vi "外观 1.vi"(0 "Data In":T5={"启动"=FALSE, "控制命令"=enum."加标回收（启动采配水）", "测量参数"={"氨氮"=TRUE, "总磷"=TRUE, "总氮"=TRUE, "CODMn"=TRUE, "CODCr"=FALSE}} caption="数据输入", 2 "Display State In":T2={"仪器状态"=FALSE, "仪器时间"=timestamp(0 s since 1904-01-01), "测量参数"={"氨氮"=TRUE, "总磷"=TRUE, "总氮"=TRUE, "CODMn"=TRUE, "CODCr"=FALSE}, "调用模块名称"="", "测试状态"={"启动时间"=timestamp(0 s since 1904-01-01), "结束时间"=timestamp(0 s since 1904-01-01), "启动次数"=0.0}} caption="显示状态输入", 3 "Container State":T4 caption="容器状态") -> (6 "Data Out":T5={"启动"=FALSE, "控制命令"=enum."加标回收（启动采配水）", "测量参数"={"氨氮"=TRUE, "总磷"=TRUE, "总氮"=TRUE, "CODMn"=TRUE, "CODCr"=FALSE}} caption="数据输出", 7 "Display State Out":T2={"仪器状态"=FALSE, "仪器时间"=timestamp(0 s since 1904-01-01), "测量参数"={"氨氮"=TRUE, "总磷"=TRUE, "总氮"=TRUE, "CODMn"=TRUE, "CODCr"=FALSE}, "调用模块名称"="", "测试状态"={"启动时间"=timestamp(0 s since 1904-01-01), "结束时间"=timestamp(0 s since 1904-01-01), "启动次数"=0.0}} caption="显示状态输出", 8 "Action":T1 caption="动作")   [LabVIEW 2016, in "ZK定时设置.xctl"]
uses:
  <vilib>/_xctls/Container State.ctl
  <vilib>/_xctls/Action.ctl
  <vilib>/_xctls/XControlSupport.lvlib
panel:
  in  "周期设置":bool
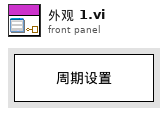
[diagram p1: front panel]
types:
  T1 = typedef "XControlSupport.lvlib/Action.ctl" = cluster{"Data Changed?":bool, "State Changed?":bool, "Action Name":string}
  T2 = typedef "ZK定时设置.xctl/状态 1.ctl" = cluster{"仪器状态":bool, "仪器时间":timestamp, "测量参数":T3, "调用模块名称":string, "测试状态":cluster{"启动时间":timestamp, "结束时间":timestamp, "启动次数":dbl}}
  T3 = typedef "ZK定时设置.xctl/测量参数.ctl" = cluster{"氨氮":bool, "总磷":bool, "总氮":bool, "CODMn":bool, "CODCr":bool}
  T4 = typedef "XControlSupport.lvlib/Container State.ctl" = cluster{"Indicator?":bool, "Run Mode?":bool, " Refnum":refnum<vi>}
  T5 = typedef "ZK定时设置.xctl/数据 1.ctl" = cluster{"启动":bool, "控制命令":T6, "测量参数":T3}
  T6 = typedef "ZK定时设置.xctl/国标控制命令.ctl" = enum16{"加标回收（启动采配水）", "加标回收（不启动采配水）", "水样测试（启动采配水）", "水样测试（不启动采配水）", "平行样测试（启动采配水）", "平行样测试（不启动采配水）", "集成干预测试"}
  T7 = cluster{"启动时间":timestamp, "结束时间":timestamp, "启动次数":dbl}
  T8 = typedef "ZK定时设置.xctl/周期模式设置.ctl" = enum16{"不启用", "定点模式", "间隔模式"}
  T9 = typedef "ZK定时设置.xctl/定点周期设置.ctl" = cluster{"启动命令":T10, "启动命令 2":T10, "启动命令 3":T10, "启动命令 4":T10, "启动命令 5":T10, "启动命令 6":T10, "启动命令 7":T10, "启动命令 8":T10, "启动命令 9":T10, "启动命令 10":T10, "启动命令 11":T10, "启动命令 12":T10, "启动命令 13":T10, "启动命令 14":T10, "启动命令 15":T10, "启动命令 16":T10, "启动命令 17":T10, "启动命令 18":T10, "启动命令 19":T10, "启动命令 20":T10, "启动命令 21":T10, "启动命令 22":T10, "启动命令 23":T10, "启动命令 24":T10}
  T10 = typedef "ZK定时设置.xctl/启动命令选择.ctl" = enum16{"", "加标回收（启动采配水）", "加标回收（不启动采配水）", "水样测试（启动采配水）", "水样测试（不启动采配水）", "平行样测试（启动采配水）", "平行样测试（不启动采配水）", "集成干预测试"}
  T11 = typedef "ZK定时设置.xctl/间隔启动设置.ctl" = cluster{"启动命令":T10, "启动间隔":dbl, "启动次数":i32}
  T12 = cluster{"周期模式":T8, "测量参数":T3, "定点周期":T9, "间隔设置":cluster{"启动命令":T10, "启动间隔":dbl, "启动次数":i32}}
  T13 = cluster{"周期模式":T8, "测量参数":T3, "定点周期":T9, "间隔启动":T11}
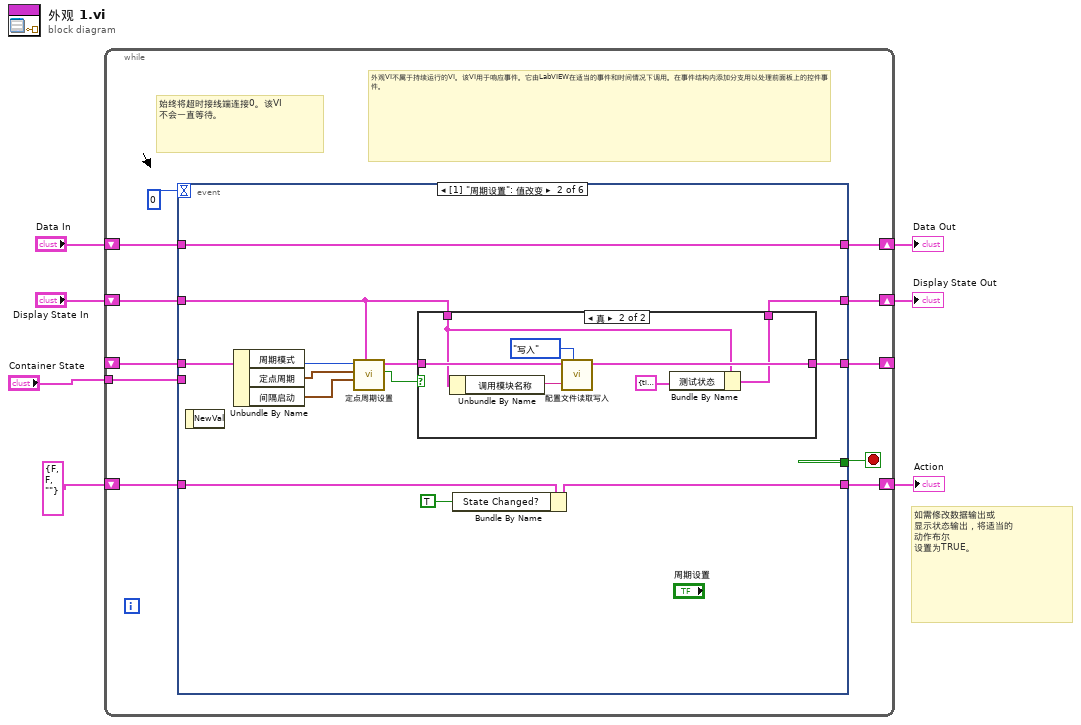
[diagram p0: block diagram]
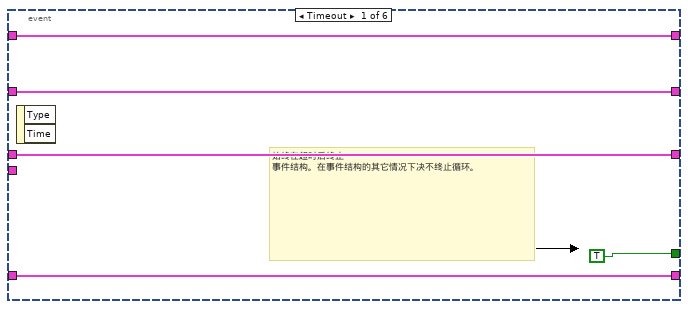
[diagram p2: hidden frame]
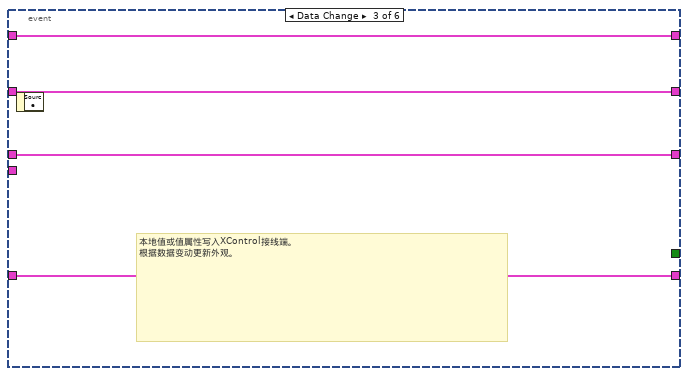
[diagram p4: hidden frame]
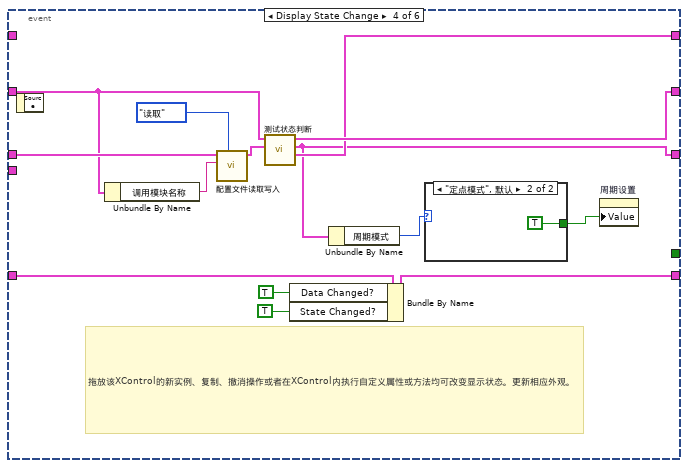
[diagram p5: hidden frame]
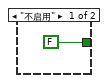
[diagram p6: hidden frame]
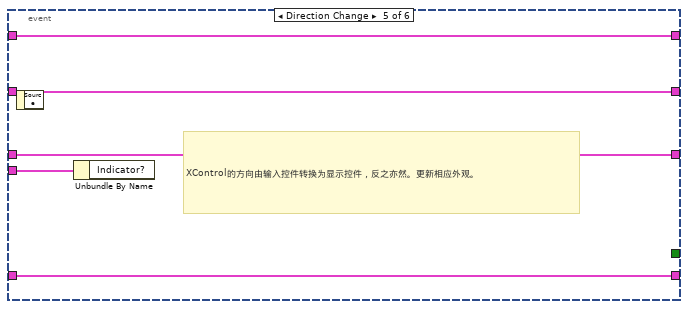
[diagram p7: hidden frame]
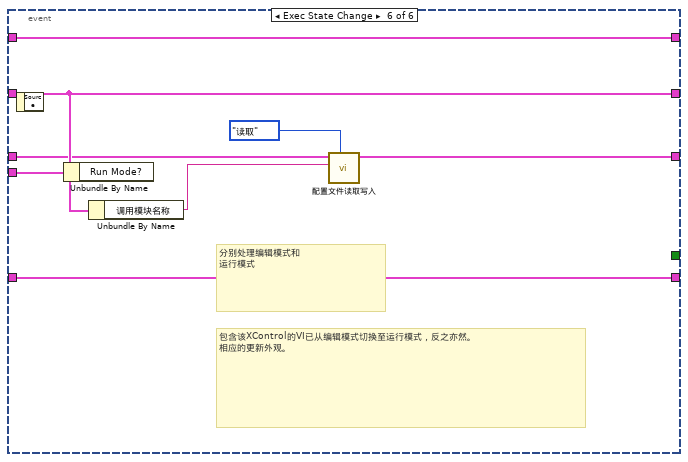
[diagram p8: hidden frame]
diagram:
  # "如需修改数据输出或\n显示状态输出，将适当的\n动作布尔\n设置为TRUE。"
  n1 = while {
    shift-right: [w17] -> w4
    shift-left: "Display State In" -> [w18]
    tunnel: "Container State" -> [w14]
    shift-right: [w12] -> w7
    shift-left: "Data In" -> [w13]
    shift-right: [w10] -> w2
    shift-left: T1 {"Data Changed?"=FALSE, "State Changed?"=FALSE, "Action Name"=""} ("Action") -> [w11]
    shift-right: [w9] -> _
    shift-left: _ -> [w8]
    stop <- w16 stop-if-true
    # "外观VI不属于持续运行的VI。该VI用于响应事件。它由LabVIEW在适当的事件和时间情况下调用。在事件结构内添加分支用以处理前面板上的控件事件。"
    # "始终将超时接线端连接0。该VI\n不会一直等待。"
    n2 = event shown="[1] \"周期设置\": 值改变" {
      selector: _ -> [_ _ _ _ _ _]
      dyn-events: _ -> [_ _ _ _ _ _]
      timeout: 0 -> [_ _ _ _ _ _]
      tunnel: w18 -> [w21 w27 w48 w57 w69 w75]
      tunnel: [w21 w26 w48 w56 w69 w75] -> w17
      tunnel: [TRUE _ _ _ _ _] -> w16
      tunnel: w14 -> [_ _ _ _ w70 w78]
      tunnel: w13 -> [w20 w36 w49 _ w68 w77]
      tunnel: [w20 w36 w49 w54 w68 w77] -> w12
      tunnel: [w22 w25 w47 w59 w67 w76] -> w10
      tunnel: w11 -> [w22 w35 w47 w63 w67 w76]
      tunnel: [w19 w29 w46 w52 w66 w72] -> w9
      tunnel: w8 -> [w19 w28 w46 w61 w66 w71]
      event Timeout {
        # "始终在超时后终止\n事件结构。在事件结构的其它情况下决不终止循环。"
        n3 = event-data() -> ()  [unwired: 1 in, 2 out]
      }
      event "周期设置": Value Change {
        n4 = event-data() -> ()  [unwired: 1 in, 1 out]
        n5 = Unbundle By Name(w28) -> ("周期模式"=w34:T8, "定点周期"=w33:T9, "间隔启动"=w32:T11)
        n6 = call "定点周期设置.vi"("Display State In"=w27, "间隔启动"=w32, "定点周期"=w33, "周期模式"=w34) -> ("保存输出"=w30:bool, "周期设置输出"=w31:T12)  [unwired: 6 in]
        n7 = case shown="真" w30 {
          tunnel: w31 -> [w38 w45]
          tunnel: w27 -> [w37 w41]
          tunnel: [w38 w42] -> w29
          tunnel: [w37 w39] -> w26
          frame False {
          }
          frame True {
            n8 = Unbundle By Name(w41) -> ("调用模块名称"=w43:string)
            n9 = call "配置文件读取写入.vi"("配置模式"=enum16{"读取", "写入"}."写入", "配置文件名"=w43, "配置信息"=w45) -> ("配置信息读取"=w42:T13)  [unwired: 7 in, 1 out]
            n10 = Bundle By Name(cluster=w41, "测试状态"=T7 {"启动时间"=timestamp(0 s since 1904-01-01), "结束时间"=timestamp(0 s since 1904-01-01), "启动次数"=0.0}) -> (w39:T2)
          }
        }
        n11 = Bundle By Name(cluster=w35, "State Changed?"=TRUE) -> (w25:T1)
      }
      event Data Change {
        # "本地值或值属性写入XControl接线端。\n根据数据变动更新外观。"
        n12 = event-data() -> ()  [unwired: 1 in, 1 out]
      }
      event Display State Change {
        # "拖放该XControl的新实例、复制、撤消操作或者在XControl内执行自定义属性或方法均可改变显示状态。更新相应外观。"
        n13 = event-data() -> ()  [unwired: 1 in, 1 out]
        n14 = Unbundle By Name(w57) -> ("调用模块名称"=w60:string)
        n15 = call "配置文件读取写入.vi"("配置模式"=enum16{"读取", "写入"}."读取", "配置文件名"=w60, "配置信息"=w61) -> ("配置信息读取"=w55:T13)  [unwired: 7 in, 1 out]
        n16 = call "测试状态判断.vi"("配置信息"=w55, "Display State In"=w57) -> ("Data In"=w54:T5, "配置信息读取"=w52:T13, "Display State Out"=w56:T2)  [unwired: 7 in]
        n17 = Bundle By Name(cluster=w63, "Data Changed?"=TRUE, "State Changed?"=TRUE) -> (w59:T1)
        n18 = Unbundle By Name(w52) -> ("周期模式"=w51:T8)
        n19 = case shown="\"定点模式\", 默认" w51 {
          tunnel: [FALSE ("周期设置") TRUE ("周期设置")] -> w50
          frame "不启用" {
          }
          frame "定点模式", Default {
          }
        }
        n20 = property on="周期设置" class="Bool (严格)"("Value"=w50) -> ()  [unwired: 2 in, 2 out]
      }
      event Direction Change {
        # "XControl的方向由输入控件转换为显示控件，反之亦然。更新相应外观。"
        n21 = event-data() -> ()  [unwired: 1 in, 1 out]
        n22 = Unbundle By Name(w70) -> ()  [unwired: 1 out]
      }
      event Exec State Change {
        # "包含该XControl的VI已从编辑模式切换至运行模式，反之亦然。\n相应的更新外观。"
        # "分别处理编辑模式和\n运行模式"
        n23 = event-data() -> ()  [unwired: 1 in, 1 out]
        n24 = Unbundle By Name(w78) -> ()  [unwired: 1 out]
        n25 = Unbundle By Name(w75) -> ("调用模块名称"=w74:string)
        n26 = call "配置文件读取写入.vi"("配置模式"=enum16{"读取", "写入"}."读取", "配置文件名"=w74, "配置信息"=w71) -> ("配置信息读取"=w72:T13)  [unwired: 7 in, 1 out]
      }
    }
  }
  "Display State Out" <- w4
  "Data Out" <- w7
  "Action" <- w2
